vi "General-Traverse.vi"(8 "error in":errorcluster, 9 "Trav Command":T1 items=["Set Reference", "Read Position", "Move", "StopMotors"], 10 "Settings":T3, 11 "Position Info IN":T2) -> (0 "error out":errorcluster, 3 "Position Info OUT":T2)   [LabVIEW 2017]
uses:
  TypeDefs/Position-Info-TD.ctl
  Settings/Settings-Control.ctl
  TypeDefs/Trav-Command-TD.ctl
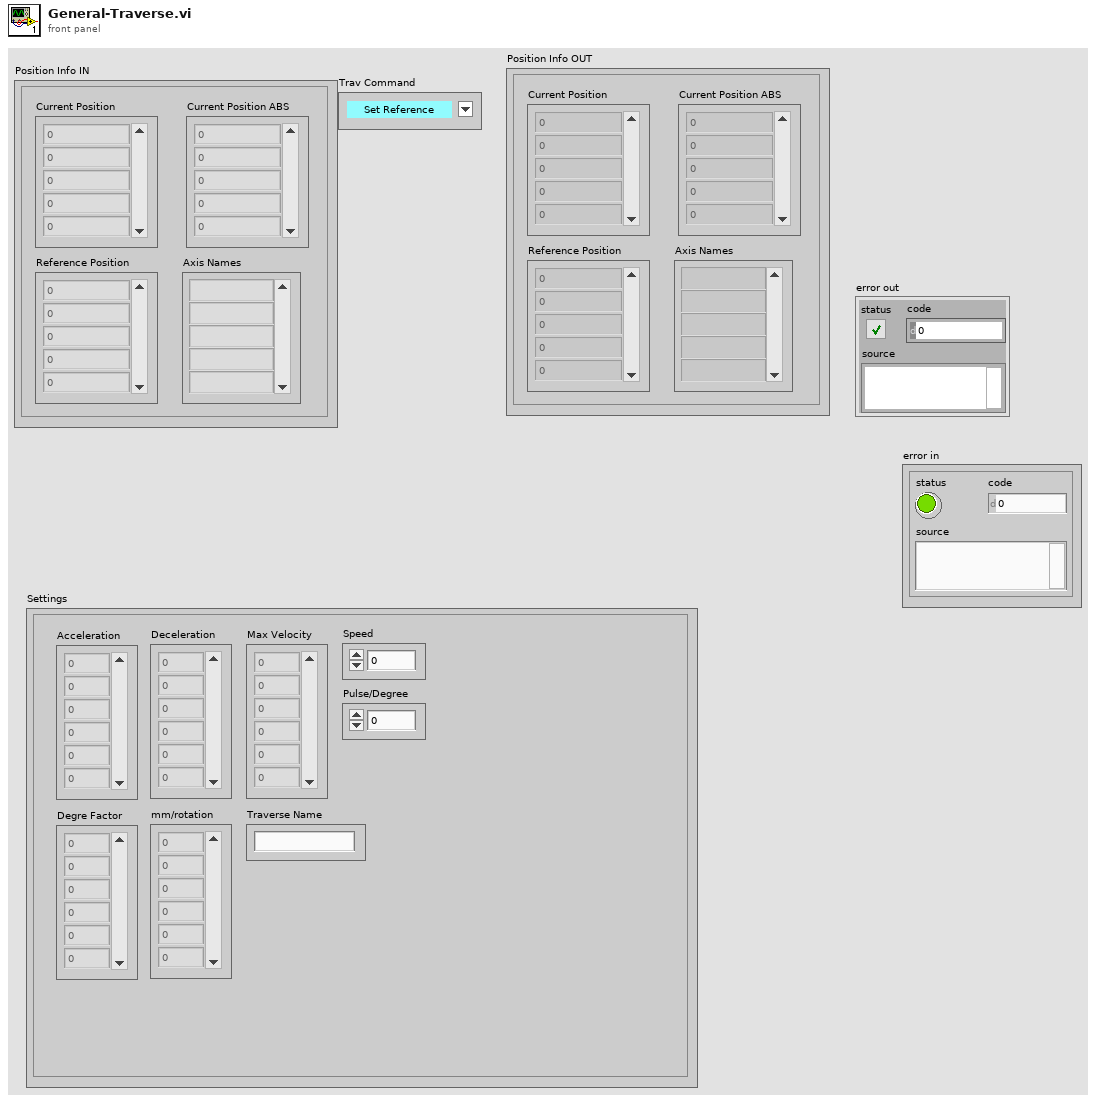
[diagram p1: front panel]
types:
  T1 = typedef "Trav-Command-TD.ctl" = u16
  T2 = typedef "Position-Info-TD.ctl" = cluster{"Current Position ABS":dbl[], "Current Position":dbl[], "Reference Position":dbl[], "Axis Names":string[]}
  T3 = typedef "Settings-Control.ctl" = cluster{"Acceleration":dbl[], "Deceleration":dbl[], "Max Velocity":dbl[], "Speed":dbl, "Pulse/Degree":dbl, "Degre Factor":dbl[], "mm/rotation":dbl[], "Traverse Name":string}
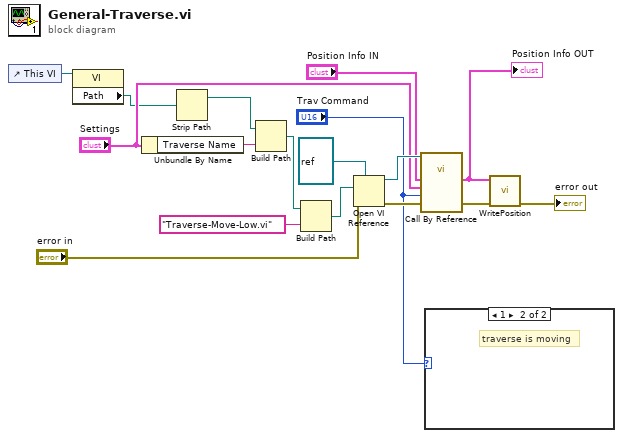
[diagram p0: block diagram]
diagram:
  n1 = control-ref of="This VI"() -> (w8:refnum<vi>)
  n2 = property class="VI"(reference=w8) -> ("Path"=w9:path)  [unwired: 1 in, 2 out]
  n3 = Unbundle By Name("Settings") -> ("Traverse Name"=w6:string)
  n4 = Strip Path(path=w9) -> (stripped path=w7:path)  [unwired: 1 out]
  n5 = Build Path(base path=w7, name or relative path=w6) -> (appended path=w5:path)
  n6 = Build Path(base path=w5, name or relative path="Traverse-Move-Low.vi") -> (appended path=w3:path)
  n7 = Open VI Reference(type specifier VI Refnum (for type only)=refnum<vi> refnum, vi path=w3, error in (no error)="error in") -> (vi reference=w16:refnum<vi>, error out=w13:errorcluster)  [unwired: 3 in]
  n8 = call-by-ref "?"(reference=w16, "error in"=w13, "Trav Command"="Trav Command", "Settings"="Settings", "Position Info IN"="Position Info IN") -> ("error out"=w12:errorcluster, "Position Info OUT"=w14:T2)  [unwired: 7 in, 2 out]
  "Position Info OUT" <- w14
  n9 = case shown="1" "Trav Command" {
    frame 0, Default {
      # "Do nothing"
    }
    frame 1 {
      # "traverse is moving"
    }
  }
  n10 = call "WritePosition.vi"("error in"=w12, "Position Info"=w14) -> ("error out"=→"error out":errorcluster)  [unwired: 9 in]
